vi "Angle Output.vi"() -> ()   [LabVIEW 2019]
panel:
  in  "Numeric":dbl
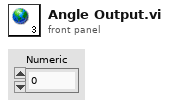
[diagram p1: front panel]
diagram:
